vi "ConfigureDlg.vi"(8 "error in (no error)":errorcluster, 11 "BaseWfrmPlugin in":refnum<class "BaseWfrmPlugin.lvclass">) -> (0 "error out":errorcluster, 3 "BaseWfrmPlugin out":refnum<class "BaseWfrmPlugin.lvclass">)   [LabVIEW 2014, in "WfrmPlugins.lvlib" / "BaseWfrmPlugin.lvclass"]
uses:
  BaseWfrmPlugin.lvclass
  TypeDefs/WfrmConfig.ctl
  BaseWfrmPlugin.lvclass/BaseWfrmPlugin.ctl
  Accessors/Write StartTime.vi
  Accessors/Write EndTime.vi
  Accessors/Write SettlingTime.vi
  Accessors/Read StartTime.vi
  Accessors/Read EndTime.vi
  Accessors/Read SettlingTime.vi
  <vilib>/Utility/config.llb/NI_LVConfig.lvlib
panel:
  in  "SettlingTime":dbl caption="Settling Time"
  in  "End Time":dbl
  in  "BtnDone":bool
  in  "StartTime":dbl caption="Start Time"
  in  "WfrmConfig":T1 caption="Waveform Configuration"
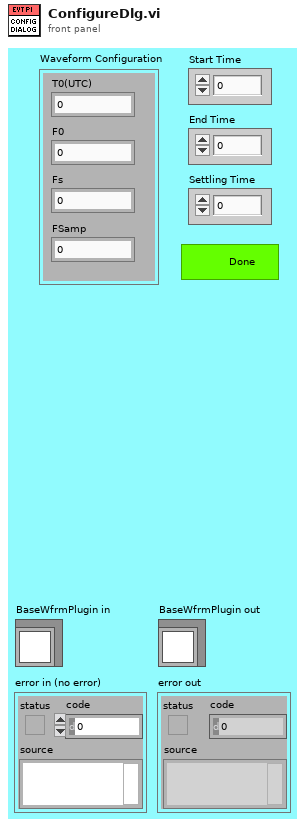
[diagram p1: front panel]
types:
  T1 = typedef "WfrmPlugins.lvlib/BaseWfrmPlugin.lvclass/WfrmConfig.ctl" = cluster{"T0(UTC)":dbl, "F0":dbl, "Fs":i32, "FSamp":u32}
  T2 = enum32{"Invalid", "Default", "Floating", "Floating/Auto-Hide", "Modal"}
  T3 = typedef "NI_LVConfig.lvlib/Config Data RefNum.ctl" = refnum<k1>
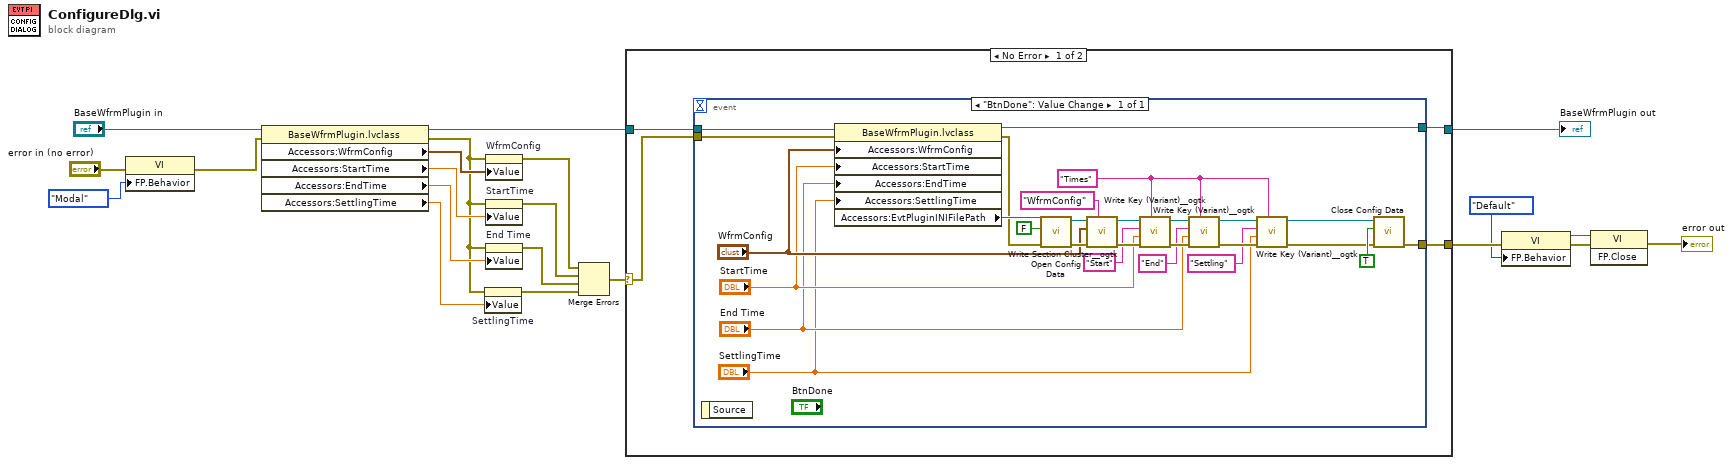
[diagram p0: block diagram]
diagram:
  n1 = property class="VI"(error in="error in (no error)", "FP.Behavior"=T2."Modal" ("Front Panel Window:Behavior")) -> (error out=w7:errorcluster)  [unwired: 1 in, 1 out]
  n2 = property class="BaseWfrmPlugin.lvclass"(reference="BaseWfrmPlugin in", error in=w7) -> (reference out=w19:refnum<class "BaseWfrmPlugin.lvclass">, error out=w14:errorcluster, "Accessors:WfrmConfig"=w18:T1, "Accessors:StartTime"=w17:dbl, "Accessors:EndTime"=w16:dbl, "Accessors:SettlingTime"=w15:dbl)
  n3 = property on="SettlingTime" class="DigNum (strict)"(error in=w14, "Value"=w15) -> (error out=w13:errorcluster)  [unwired: 1 in, 1 out]
  n4 = property on="WfrmConfig" class="Clust (strict)"(error in=w14, "Value"=w18) -> (error out=w11:errorcluster)  [unwired: 1 in, 1 out]
  n5 = property on="StartTime" class="DigNum (strict)"(error in=w14, "Value"=w17) -> (error out=w10:errorcluster)  [unwired: 1 in, 1 out]
  n6 = property on="End Time" class="DigNum (strict)"(error in=w14, "Value"=w16) -> (error out=w9:errorcluster)  [unwired: 1 in, 1 out]
  n7 = Merge Errors(w11, w10, w9, w13) -> (w8:errorcluster)
  n8 = case shown="No Error" w8 {
    selector: w8 -> [w24 w54]
    tunnel: [w22 w54] -> w5
    tunnel: [w23 w53] -> w20
    tunnel: w19 -> [w25 w53]
    frame No Error {
      n9 = event shown="[0] \"BtnDone\": Value Change" {
        selector: _ -> [_]
        dyn-events: _ -> [_]
        timeout: _ -> [_]
        tunnel: w25 -> [w52]
        tunnel: w24 -> [w49]
        tunnel: [w40] -> w22
        tunnel: [w39] -> w23
        event "BtnDone": Value Change {
          w26 = "Times"
          n10 = event-data() -> ()  [unwired: 1 in, 1 out]
          n11 = property class="BaseWfrmPlugin.lvclass"(reference=w52, error in=w49, "Accessors:WfrmConfig"="WfrmConfig", "Accessors:StartTime"="StartTime", "Accessors:EndTime"="End Time", "Accessors:SettlingTime"="SettlingTime") -> (reference out=w39:refnum<class "BaseWfrmPlugin.lvclass">, error out=w48:errorcluster, "Accessors:EvtPluginINIFilePath"=w51:path)
          n12 = call <vilib>:"Open Config Data.vi"("error in (no error)"=w48, "create file if necessary (T)"=FALSE, "configuration file path"=w51) -> ("error out"=w47:errorcluster, "refnum"=w46:T3)  [unwired: 6 in, 1 out]
          n13 = call <userlib>:"Write Section Cluster__ogtk.vi"("section (optional)"="WfrmConfig", "error in (no error)"=w47, "Section Formatted Cluster"="WfrmConfig", "refnum"=w46) -> ("error out"=w43:errorcluster, "dup refnum"=w42:T3)  [unwired: 6 in]
          n14 = call <userlib>:"Write Key (Variant)__ogtk.vi"("section"=w26, "error in (no error)"=w43, "key-value"="StartTime", "key (optional)"="Start", "refnum"=w42) -> ("error out"=w38:errorcluster, "refnum out"=w37:T3)  [unwired: 5 in]
          n15 = call <userlib>:"Write Key (Variant)__ogtk.vi"("section"=w26, "error in (no error)"=w38, "key-value"="End Time", "key (optional)"="End", "refnum"=w37) -> ("error out"=w36:errorcluster, "refnum out"=w35:T3)  [unwired: 5 in]
          n16 = call <userlib>:"Write Key (Variant)__ogtk.vi"("section"=w26, "error in (no error)"=w36, "key-value"="SettlingTime", "key (optional)"="Settling", "refnum"=w35) -> ("error out"=w28:errorcluster, "refnum out"=w27:T3)  [unwired: 5 in]
          n17 = call <vilib>:"Close Config Data.vi"("error in (no error)"=w28, "write file if changed (T)"=TRUE, "refnum"=w27) -> ("error out"=w40:errorcluster)  [unwired: 7 in, 1 out]
        }
      }
    }
    frame Error {
    }
  }
  "BaseWfrmPlugin out" <- w20
  n18 = property class="VI"(error in=w5, "FP.Behavior"=T2."Default" ("Front Panel Window:Behavior")) -> (reference out=w2:refnum<vi>, error out=w3:errorcluster)  [unwired: 1 in]
  n19 = invoke class="VI" method="FP.Close"(reference=w2, error in=w3) -> (error out=→"error out":errorcluster)  [unwired: 1 in, 2 out]
